vi "FTS Get Instrument Property PD_tempVariable.vi"(8 "error in (no error)":errorcluster, 10 "channel":u16, 11 "spectrIdx":u16) -> (0 "error out":errorcluster, 2 "tempVar_available":bool)   [LabVIEW 2010, in "FTSLib.lvlib"]
uses:
  FTSLib.lvlib
  FTSLib.dll
panel:
  out "return type":u8
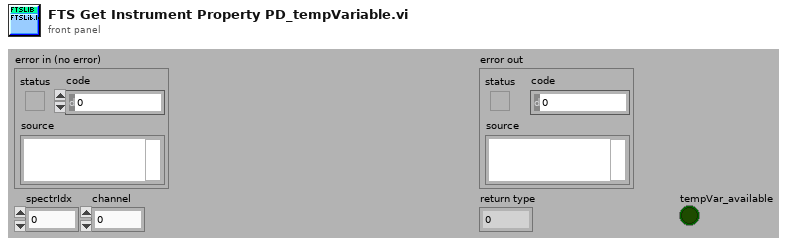
[diagram p1: front panel]
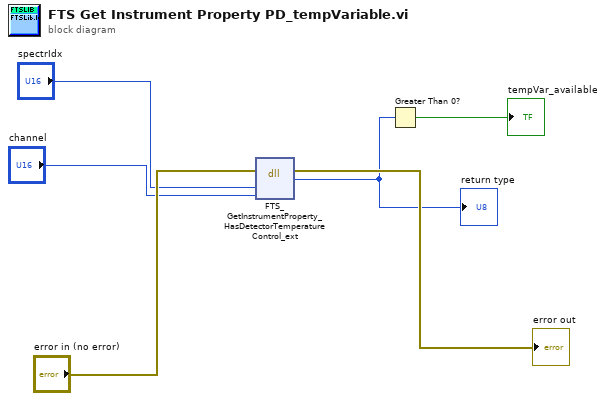
[diagram p0: block diagram]
diagram:
  n1 = dll-call lib="FTSLib.dll" fn="FTS_GetInstrumentProperty_HasDetectorTemperatureControl_ext"(error in="error in (no error)", "spectrIdx"="spectrIdx", "channel"="channel") -> (error out=→"error out":errorcluster, "return type"=w2:u8)  [unwired: 4 in, 1 out]
  "return type" <- w2
  n2 = Greater Than 0?(x=w2) -> (x > 0?=→"tempVar_available":bool)
